vi "JSR_Control_Enumerator.vi"(8 "Voltage (V) Ref":refnum<vi>, 9 "Gain (db) Ref":refnum<vi>, 10 "Pulse Energy Level Ref":refnum<vi>) -> (1 "Voltage":T1, 2 "Gain":T1, 3 "Pulse Energy Level":T1)   [LabVIEW 2022 SP3]
uses:
  <vilib>/Utility/miscctls.llb/LVStringsAndValuesArrayTypeDef_U16.ctl
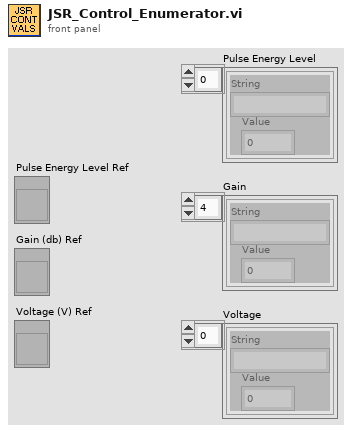
[diagram p1: front panel]
types:
  T1 = typedef "LVStringsAndValuesArrayTypeDef_U16.ctl" = cluster{"String":string, "Value":u16}[]
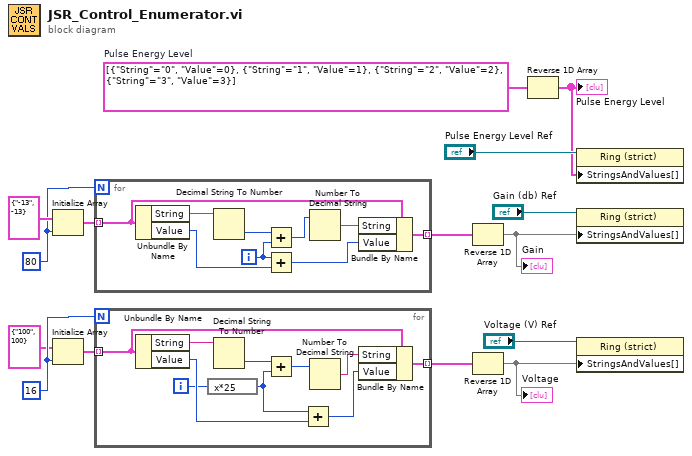
[diagram p0: block diagram]
diagram:
  w6 = 16
  w9 = 80
  w11 = T1 [{"String"="0", "Value"=0}, {"String"="1", "Value"=1}, {"String"="2", "Value"=2}, {"String"="3", "Value"=3}]  # Pulse Energy Level
  n1 = Initialize Array(cluster{"String":string, "Value":i32} {"String"="-13", "Value"=-13}, w9) -> (w8:cluster{"String":string, "Value":i32}[])
  n2 = Initialize Array(cluster{"String":string, "Value":i32} {"String"="100", "Value"=100}, w6) -> (w7:cluster{"String":string, "Value":i32}[])
  n3 = for {
    N: w9 -> [_]
    tunnel: w8 -> [w24] mode=indexing
    tunnel: [w16] -> w3 mode=indexing
    i -> [w17]
    n4 = Unbundle By Name(w24) -> ("String"=w21:string, "Value"=w23:i32)
    n5 = Decimal String To Number(string=w21) -> (number=w19:i32)  [unwired: 2 in, 1 out]
    n6 = Add(x=w19, y=w17) -> (x+y=w18:i32)
    n7 = Add(x=w17, y=w23) -> (x+y=w22:i32)
    n8 = Number To Decimal String(number=w18) -> (decimal integer string=w20:string)  [unwired: 1 in]
    n9 = Bundle By Name(cluster=w24, "String"=w20, "Value"=w22) -> (w16:cluster{"String":string, "Value":i32})
  }
  n10 = for {
    N: w6 -> [_]
    tunnel: w7 -> [w34] mode=indexing
    tunnel: [w26] -> w2 mode=indexing
    i -> [w27]
    n11 = Unbundle By Name(w34) -> ("String"=w31:string, "Value"=w33:i32)
    n12 = expression code="x*25"(w27) -> (w25:i32)
    n13 = Decimal String To Number(string=w31) -> (number=w29:i32)  [unwired: 2 in, 1 out]
    n14 = Add(x=w29, y=w25) -> (x+y=w28:i32)
    n15 = Add(x=w25, y=w33) -> (x+y=w32:i32)
    n16 = Number To Decimal String(number=w28) -> (decimal integer string=w30:string)  [unwired: 1 in]
    n17 = Bundle By Name(cluster=w34, "String"=w30, "Value"=w32) -> (w26:cluster{"String":string, "Value":i32})
  }
  n18 = Reverse 1D Array(array=w3) -> (reversed array=w4:cluster{"String":string, "Value":i32}[])
  "Gain" <- w4
  n19 = Reverse 1D Array(array=w2) -> (reversed array=w1:cluster{"String":string, "Value":i32}[])
  "Voltage" <- w1
  n20 = Reverse 1D Array(array=w11) -> (reversed array=w12:T1)
  "Pulse Energy Level" <- w12
  n21 = property class="Ring (strict)"(reference="Pulse Energy Level Ref", "StringsAndValues[]"=w12) -> ()  [unwired: 1 in, 2 out]
  n22 = property class="Ring (strict)"(reference="Gain (db) Ref", "StringsAndValues[]"=w4) -> ()  [unwired: 1 in, 2 out]
  n23 = property class="Ring (strict)"(reference="Voltage (V) Ref", "StringsAndValues[]"=w1) -> ()  [unwired: 1 in, 2 out]
